vi "Fluke 884X Series Read Math Measurements.vi"() -> ()   [LabVIEW 2010]
doc: "This example shows how to configure a Math measurement and take multiple readings."
uses:
  <vilib>/Utility/error.llb/DialogType.ctl
  <instrlib>/Fluke 884X Series/Public/Data/Read (Multiple Points).vi
  <instrlib>/Fluke 884X Series/Fluke 884X Series.lvlib
panel:
  out "Measurements":dbl[](array[numeric])
  out "Average":dbl
  out "Minimum":dbl
  out "Maximum":dbl
  in  "Function (0: DC Voltage)":u16(ring) items=["DC Voltage", "AC Voltage", "2 - Wire Resistance", "4 - Wire Resistance", "DC Current", "AC Current", "Frequency", "Period", "Continuity", "Diode Checking", "Temperature", "Capacitance"]
  in  "Serial Configuration":T1={"Baud Rate"=9600, "Parity"=0, "Data Bits"=8, "Stop Bits"=10, "Flow Control"=0} {"Flow Control" items=["None", "XON/XOFF", "RTS/CTS", "XON/XOFF & RTS/CTS", "DTR/DSR", "XON/XOFF & DTR/DSR"]; "Stop Bits" items=["1.0"=10, "1.5"=15, "2.0"=20]; "Data Bits" items=["7"=7, "8"=8]; "Parity" items=["None", "Odd", "Even", "Mark", "Space"]; "Baud Rate" items=["300"=300, "600"=600, "1200"=1200, "2400"=2400, "4800"=4800, "9600"=9600, "19200"=19200]}
  in  "VISA resource name":refnum<visa-resource-name>
  # "(c) 2007 National Instruments.  ALL RIGHTS RESERVED."
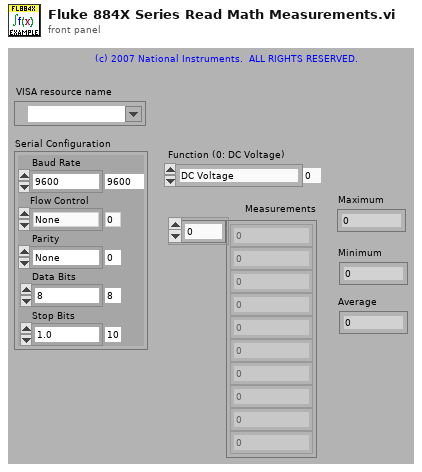
[diagram p1: front panel]
types:
  T1 = cluster{"Baud Rate":u32, "Parity":u16, "Data Bits":u16, "Stop Bits":u16, "Flow Control":u16}
  T2 = enum16{"None", "Min/Max", "Null", "dB", "dBm", "Limit"}
  T3 = typedef "DialogType.ctl" = u16
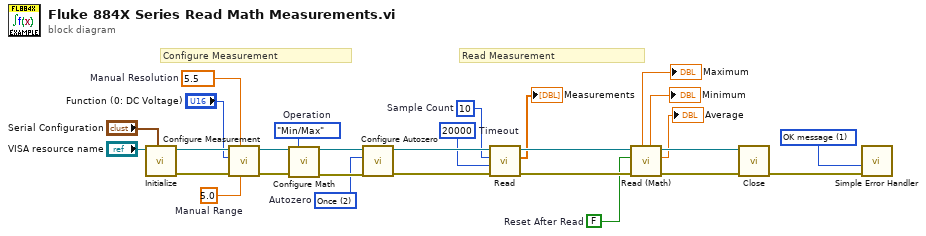
[diagram p0: block diagram]
diagram:
  w1 = 5.0  # Manual Range
  w2 = 5.5 items=["4.5"=4.5, "5.5"=5.5, "6.5"=6.5]  # Manual Resolution
  w7 = FALSE  # Reset After Read
  w8 = 20000  # Timeout
  w9 = 10  # Sample Count
  w10 = u16 2 items=["On", "Off", "Once"]  # Autozero
  w11 = T2."Min/Max"  # Operation
  w15 = T3 1 items=["no dialog", "OK message", "continue or stop message", "OK message + warnings", "continue/stop + warnings"] ("type of dialog (OK msg:1)")
  # "Read Measurement"
  # "Configure Measurement"
  n1 = call <instrlib>:"Initialize.vi"("Serial Configuration"="Serial Configuration", "VISA resource name"="VISA resource name") -> ("error out"=w26:errorcluster, "VISA resource name out"=w27:refnum<visa-resource-name>)  [unwired: 8 in]
  n2 = call <instrlib>:"Configure Measurement.vi"("Manual Range (1.0)"=w1, "Manual Resolution (5.5 Digits)"=w2, "error in (no error)"=w26, "Function (0: DC Voltage)"="Function (0: DC Voltage)", "VISA resource name"=w27) -> ("error out"=w22:errorcluster, "VISA resource name out"=w23:refnum<visa-resource-name>)  [unwired: 5 in]
  n3 = call <instrlib>:"Configure Math.vi"("VISA resource name"=w23, "Operation (0:None)"=w11, "error in (no error)"=w22) -> ("VISA resource name out"=w21:refnum<visa-resource-name>, "error out"=w20:errorcluster)  [unwired: 11 in]
  n4 = call <instrlib>:"Configure Autozero.vi"("error in (no error)"=w20, "Autozero  (0: On)"=w10, "VISA resource name"=w21) -> ("error out"=w24:errorcluster, "VISA resource name out"=w25:refnum<visa-resource-name>)  [unwired: 7 in]
  n5 = call-poly <instrlib>:"Read.vi"("error in (no error)"=w24, "Timeout (10000 ms)"=w8, "Sample Count (1)"=w9, "VISA resource name"=w25) -> ("error out"=w18:errorcluster, "Measurements"=→"Measurements":dbl[], "VISA resource name out"=w19:refnum<visa-resource-name>)  [unwired: 5 in]
  n6 = call <instrlib>:"Read (Math).vi"("error in (no error)"=w18, "Reset After Read (False)"=w7, "VISA resource name"=w19) -> ("error out"=w16:errorcluster, "Average"=→"Average":dbl, "VISA resource name out"=w17:refnum<visa-resource-name>, "Minimum"=→"Minimum":dbl, "Maximum"=→"Maximum":dbl)  [unwired: 3 in, 1 out]
  n7 = call <instrlib>:"Close.vi"("error in (no error)"=w16, "VISA resource name"=w17) -> ("error out"=w28:errorcluster)  [unwired: 9 in]
  n8 = call <vilib>:"Simple Error Handler.vi"("type of dialog (OK msg:1)"=w15, "error in (no error)"=w28) -> ()  [unwired: 3 in, 5 out]
